vi "TEST DEBUG.vi"() -> ()   [LabVIEW 2011]
panel:
  out "Debugging 2?":bool
  in  "stop":bool
  out "running":bool
  out "Debugging 1?":bool
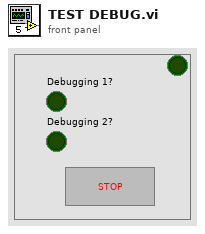
[diagram p1: front panel]
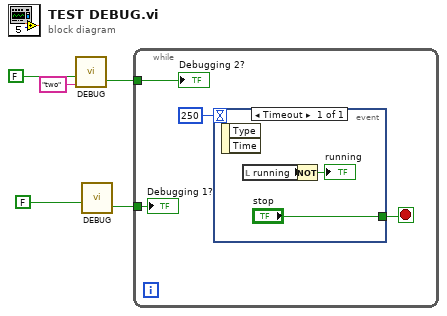
[diagram p0: block diagram]
diagram:
  n1 = call "DEBUG.vi"("Debug Tag (none)"="two", "Dev DEBUG? (f)"=FALSE) -> ("DEBUG?"=w3:bool)  [unwired: 3 in]
  n2 = call "DEBUG.vi"("Dev DEBUG? (f)"=FALSE) -> ("DEBUG?"=w5:bool)  [unwired: 4 in]
  n3 = while {
    tunnel: w5 -> [w7]
    tunnel: w3 -> [w6]
    stop <- w9 stop-if-true
    n4 = event shown="[0] Timeout" {
      selector: _ -> [_]
      dyn-events: _ -> [_]
      timeout: 250 -> [_]
      tunnel: ["stop"] -> w9
      event Timeout {
        n5 = event-data() -> ()  [unwired: 1 in, 2 out]
        n6 = local read "running"() -> (w11:bool)
        n7 = Not(x=w11) -> (.not. x?=→"running":bool)
      }
    }
    "Debugging 1?" <- w7
    "Debugging 2?" <- w6
  }
